vi "ILC Physical Learning.vi"(6 "PID Cluster":T6={"L1 to L4 PID Cluster"={"L1 PID Gains"={"Kp"=0.005, "Kd"=0.5, "Ki"=0.0005}, "L2 PID Gains"={"Kp"=0.01, "Kd"=1.0, "Ki"=0.005}, "L3 PID Gains"={"Kp"=0.05, "Kd"=1.0, "Ki"=0.0005}, "L4 PID Gains"={"Kp"=0.1, "Kd"=0.1, "Ki"=0.0005}}, "Stage PID Cluster"={"Stage Z PID"={"Kp"=0.0005, "Kd"=0.001, "Ki"=0.0}, "Stage Y PID"={"Kp"=0.0003, "Kd"=0.01, "Ki"=0.0}, "Stage X PID"={"Kp"=0.0003, "Kd"=0.01, "Ki"=0.0}}, "OCT Z PID Gains"={"Kp"=0.0003, "Kd"=0.0001, "Ki"=0.01}}, 8 "error in":errorcluster, 9 "Offset Home 2 RCM":dbl[](array[numeric])=[0.0, 0.0, 0.0, 0.0], 10 "Prev Posit Cluster":T5={"Prev L1 to L4 Posit"=[-0.5319, -0.035669172703475985, -2.0566170657346783, 0.9099264705882353], "Prev Stage Posit"=[6.002553885707208, 5.996566124542428, 5.995469940427586], "Prev OCT Z Posit"=-0.0}, 11 "FPGA VI Reference In":refnum<k20>) -> (0 "Eye Model Cluster":T3={"X Grid"=[], "Y Grid"=[], "Za_true Surf"=[], "Iris Center"=[0.0, 5.0, 0.0], "Zp_true Surf"=[], "Pinv"=[[1.0, 0.0], [0.0, 1.0]], "za_true"=0.0, "za_work"=0.0, "zp_work"=0.0, "zp_true"=0.0}, 1 "Trajectory Cluster":T1, 2 "Last Posit Cluster":T4={"Last L1 to L4 Posit"=[0.0, 0.0, 0.0, 0.0], "Last Stage Posit"=[6.0, 6.0, 6.0], "Last OCT Z Posit"=0.0}, 3 "FPGA VI Reference Out":refnum<k20>, 4 "error out":errorcluster, 5 "First Trk Pt":dbl[](array[numeric]))   [LabVIEW 2016]
uses:
  <vilib>/Analysis/Matrix/Datatypes/RealMatrix.ctl
  <vilib>/Platform/TimedLoop/XDataNode/timing_clust.ctl
  <vilib>/Platform/TimedLoop/XDataNode/nitl_modes.ctl
  <vilib>/Platform/TimedLoop/XDataNode/wakeup.ctl
  Global Variables.vi
  <vilib>/platform/TimedLoop/XDataNode/XDataNode.xnode
  <vilib>/Platform/TimedLoop/XDataNode/XDNodeRunTimeDep.lvlib
  <vilib>/Analysis/Matrix/NI_Matrix.lvlib
panel:
  out "In Servo Loop":bool
  out "Loading Finished":bool
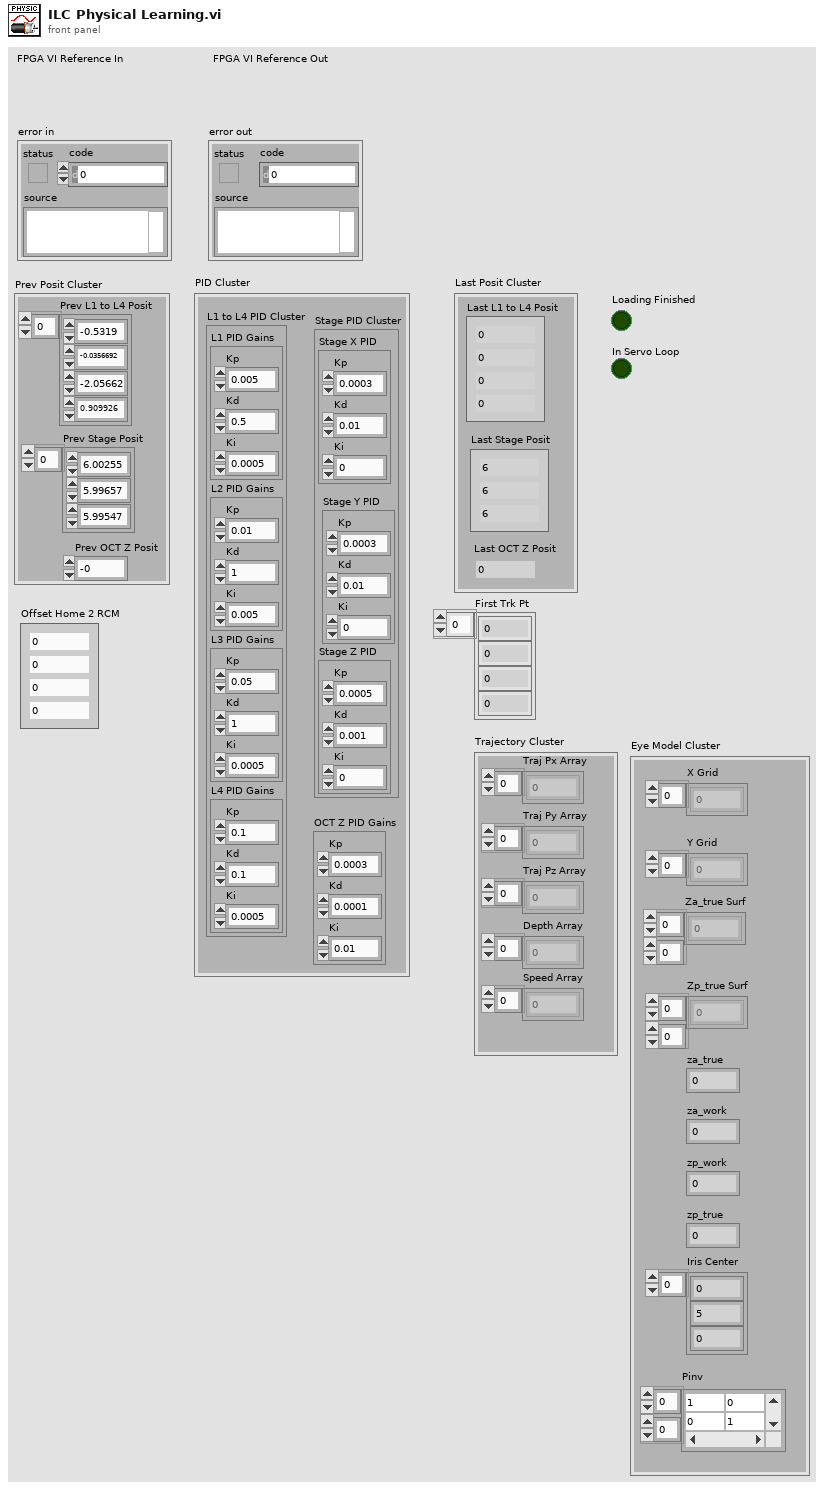
[diagram p1: front panel]
types:
  T1 = cluster{"Traj Px Array":dbl[], "Traj Py Array":dbl[], "Traj Pz Array":dbl[], "Speed Array":dbl[], "Depth Array":dbl[]}
  T2 = typedef "NI_Matrix.lvlib/RealMatrix.ctl" = dbl[][]
  T3 = cluster{"X Grid":dbl[], "Y Grid":dbl[], "Za_true Surf":dbl[][], "Iris Center":dbl[], "Zp_true Surf":dbl[][], "Pinv":T2, "za_true":dbl, "za_work":dbl, "zp_work":dbl, "zp_true":dbl}
  T4 = cluster{"Last L1 to L4 Posit":dbl[], "Last Stage Posit":dbl[], "Last OCT Z Posit":dbl}
  T5 = cluster{"Prev L1 to L4 Posit":dbl[], "Prev Stage Posit":dbl[], "Prev OCT Z Posit":dbl}
  T6 = cluster{"L1 to L4 PID Cluster":cluster{"L1 PID Gains":cluster{"Kp":dbl, "Kd":dbl, "Ki":dbl}, "L2 PID Gains":cluster{"Kp":dbl, "Kd":dbl, "Ki":dbl}, "L3 PID Gains":cluster{"Kp":dbl, "Kd":dbl, "Ki":dbl}, "L4 PID Gains":cluster{"Kp":dbl, "Kd":dbl, "Ki":dbl}}, "Stage PID Cluster":cluster{"Stage Z PID":cluster{"Kp":dbl, "Kd":dbl, "Ki":dbl}, "Stage Y PID":cluster{"Kp":dbl, "Kd":dbl, "Ki":dbl}, "Stage X PID":cluster{"Kp":dbl, "Kd":dbl, "Ki":dbl}}, "OCT Z PID Gains":cluster{"Kp":dbl, "Kd":dbl, "Ki":dbl}}
  T7 = typedef "XDNodeRunTimeDep.lvlib/timing_clust.ctl" = cluster{"Expected End [f-1]":u64, "Actual End [f-1]":u64, "Finished Late? [f-1]":bool, "Expected End [i-1]":u64, "Actual End [i-1]":u64, "Finished Late? [i-1]":bool, "Expected Start [i]":u64, "Actual Start [i]":u64, "Expected Start [f]":u64, "Actual Start [f]":u64, "Source Name":string, "Structure Name":string, "Period":i64, "Deadline":i64, "Offset":i64, "Start":i64, "Priority":i32, "Timeout":i32, "Mode":T8, "Wakeup Reason":T9, "Error":errorcluster, "Source Type":string, "Secondary Source Type":string, "Global End Time":u64, "Global Start Time":u64, "Frame Duration":u64, "Iteration Duration":u64, "Assigned CPU":i32, "I/O Scan Engine Mode":u32}
  T8 = typedef "XDNodeRunTimeDep.lvlib/nitl_modes.ctl" = enum32{"No Change", "Process missed periods, maintain original phase", "Discard missed periods, maintain original phase", "Process missed periods, ignore original phase", "Discard missed periods, ignore original phase"}
  T9 = typedef "XDNodeRunTimeDep.lvlib/wakeup.ctl" = enum32{"Normal", "Aborted", "Asynchronous wakeup", "Timing source error", "Timed loop error", "Timeout"}
  T10 = cluster{"Stop Vacuum":bool, "Vacuum Force":i8, "Max Limit [mmHg]":dbl, "Slide in":i8, "Irrigation?":bool}
  T11 = cluster{"L1 PID Gains":cluster{"Kp":dbl, "Kd":dbl, "Ki":dbl}, "L2 PID Gains":cluster{"Kp":dbl, "Kd":dbl, "Ki":dbl}, "L3 PID Gains":cluster{"Kp":dbl, "Kd":dbl, "Ki":dbl}, "L4 PID Gains":cluster{"Kp":dbl, "Kd":dbl, "Ki":dbl}}
  T12 = cluster{"Stage Z PID":cluster{"Kp":dbl, "Kd":dbl, "Ki":dbl}, "Stage Y PID":cluster{"Kp":dbl, "Kd":dbl, "Ki":dbl}, "Stage X PID":cluster{"Kp":dbl, "Kd":dbl, "Ki":dbl}}
  T13 = cluster{"Accurus button":bool[], "Accurus engaged?":bool, "Vacuum Force":i32, "Accurus Ch. A Vout":dbl, "Accurus Ch. B Vout":dbl, "Irrigation engaged?":bool}
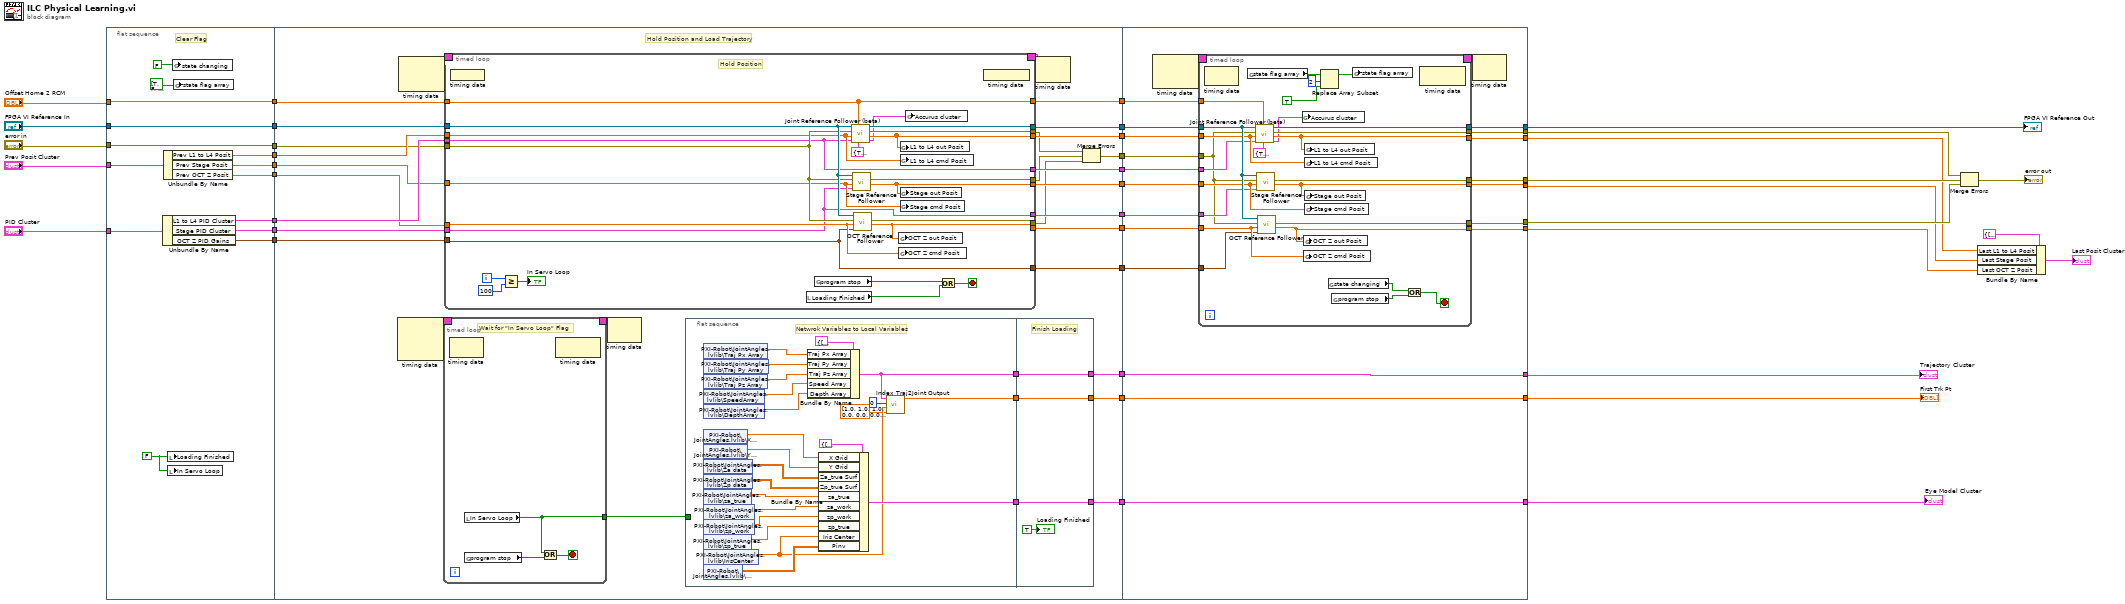
[diagram p0: block diagram]
diagram:
  n1 = flat-sequence {
    tunnel: [w51] -> w39
    tunnel: "FPGA VI Reference In" -> [w51]
    tunnel: [w50] -> w37
    tunnel: "error in" -> [w50]
    tunnel: "Prev Posit Cluster" -> [w49]
    tunnel: "PID Cluster" -> [w48]
    tunnel: [w47] -> w35
    tunnel: [w46] -> w34
    tunnel: "Offset Home 2 RCM" -> [w45]
    tunnel: [w45] -> w32
    tunnel: [w44] -> w29
    tunnel: [w43] -> w28
    tunnel: [w42] -> w27
    tunnel: [w41] -> w26
    tunnel: w39 -> [w68]
    tunnel: w37 -> [w63]
    tunnel: w35 -> [w65]
    tunnel: w34 -> [w64]
    tunnel: w32 -> [w69]
    tunnel: w29 -> [w67]
    tunnel: w28 -> [w62]
    tunnel: w27 -> [w61]
    tunnel: w26 -> [w66]
    tunnel: [w85] -> w13
    tunnel: [w84] -> w12
    tunnel: [w83] -> w11
    tunnel: [w82] -> w10
    tunnel: [w81] -> w9
    tunnel: [w80] -> w8
    tunnel: [w79] -> w7
    tunnel: [w78] -> w6
    tunnel: [w77] -> w5
    tunnel: [w57] -> w4
    tunnel: [w56] -> w3
    tunnel: [w54] -> w2
    tunnel: w13 -> [w165]
    tunnel: [w164] -> w24
    tunnel: [w163] -> w23
    tunnel: [w162] -> w22
    tunnel: w12 -> [w161]
    tunnel: w11 -> [w160]
    tunnel: w10 -> [w159]
    tunnel: w9 -> [w158]
    tunnel: w8 -> [w157]
    tunnel: w7 -> [w156]
    tunnel: w6 -> [w155]
    tunnel: [w154] -> w20
    tunnel: [w153] -> w19
    tunnel: [w152] -> w18
    tunnel: [w151] -> w16
    tunnel: [w148] -> w14
    tunnel: w5 -> [w150]
    tunnel: [w150] -> w15
    tunnel: w4 -> [w149]
    tunnel: w3 -> [w148]
    tunnel: [w147] -> w1
    tunnel: w2 -> [w147]
    frame #0 {
      w40 = FALSE ("Loading Finished")
      # "Clear Flag"
      n2 = Unbundle By Name(w48) -> ("L1 to L4 PID Cluster"=w46:T11, "Stage PID Cluster"=w47:T12, "OCT Z PID Gains"=w41:cluster{"Kp":dbl, "Kd":dbl, "Ki":dbl})
      n3 = Unbundle By Name(w49) -> ("Prev L1 to L4 Posit"=w44:dbl[], "Prev Stage Posit"=w43:dbl[], "Prev OCT Z Posit"=w42:dbl)
      n4 = local write "Loading Finished"(w40) -> ()
      n5 = local write "In Servo Loop"(w40) -> ()
      n6 = global write "Global Variables.vi" "state changing"(FALSE ("state changing")) -> ()
      n7 = global write "Global Variables.vi" "state flag array"(bool[] [TRUE, FALSE, FALSE, FALSE, FALSE, FALSE, FALSE, FALSE, FALSE] ("state flag array")) -> ()
    }
    frame #1 {
      # "Hold Position and Load Trajectory"
      n8 = node-c288() -> (w72:T7)  [unwired: 3 in]
      n9 = node-c288() -> (w76:T7)  [unwired: 2 in]
      n10 = timed-loop {
        timing: w72 -> [_]
        timing-out: [_] -> w71
        tunnel: [w87] -> w70
        stop <- w88 stop-if-true
        # "Wait for \"In Servo Loop\" Flag"
        n11 = node-c288() -> ()  [unwired: 1 in, 1 out]
        n12 = local read "In Servo Loop"() -> (w87:bool)
        n13 = global read "Global Variables.vi" "program stop"() -> (w86:bool)
        n14 = Or(x=w87, y=w86) -> (x .or. y?=w88:bool)
        n15 = node-c288() -> ()  [unwired: 1 in, 1 out]
      }
      n16 = timed-loop {
        timing: w76 -> [_]
        timing-out: [_] -> w75
        tunnel: w67 -> [w136]
        tunnel: w62 -> [w134]
        tunnel: w65 -> [w124]
        tunnel: w64 -> [w125]
        tunnel: w63 -> [w138]
        tunnel: w68 -> [w139]
        tunnel: w69 -> [w131]
        tunnel: w61 -> [w132]
        tunnel: w66 -> [w126]
        tunnel: [w137] -> w83
        tunnel: [w135] -> w82
        tunnel: [w133] -> w81
        tunnel: [w131] -> w84
        tunnel: [w130] -> w85
        tunnel: [w129] -> w60
        tunnel: [w128] -> w59
        tunnel: [w127] -> w58
        tunnel: [w126] -> w80
        tunnel: [w125] -> w79
        tunnel: [w124] -> w78
        i -> [w123]
        stop <- w142 stop-if-true
        # "Hold Position"
        n17 = node-c288 ("Output Node")() -> ()  [unwired: 1 in]
        n18 = Greater Or Equal?(x=w123, y=100) -> (x >= y?=→"In Servo Loop":bool)
        n19 = local read "Loading Finished"() -> (w141:bool)
        n20 = global read "Global Variables.vi" "program stop"() -> (w140:bool)
        n21 = call "Joint Reference Follower (beta).vi"("Accurus Ctrl Cluster"=T10 {"Stop Vacuum"=TRUE, "Vacuum Force"=0, "Max Limit [mmHg]"=600.0, "Slide in"=0, "Irrigation?"=TRUE}, "Offset Home2RCM [deg/mm]"=w131, "PID Ctrl Cluster"=w125, "Ref Array [deg/mm]"=w136, "error in"=w138, "FPGA VI Reference In"=w139) -> ("Accurus Output Cluster"=w119:T13, "Output Posit Array [deg/mm]"=w137:dbl[], "error out"=w129:errorcluster, "FPGA VI Reference Out"=w130:refnum<k20>)  [unwired: 2 in]
        n22 = call "Stage Reference Follower.vi"("Stage PID Cluster"=w124, "Stage cmd Posit [mm]"=w134, "error in"=w138, "FPGA VI Reference In"=w139) -> ("Stage out Posit [mm]"=w135:dbl[], "error out"=w128:errorcluster)  [unwired: 5 in, 1 out]
        n23 = call "OCT Reference Follower.vi"("OCT Z PID Gains"=w126, "OCT  Z cmd Posit [mm]"=w132, "error in"=w138, "FPGA VI Reference In"=w139) -> ("OCT  Z out Posit [mm]"=w133:dbl, "error out"=w127:errorcluster)  [unwired: 5 in, 1 out]
        n24 = global write "Global Variables.vi" "OCT Z out Posit"(w133) -> ()
        n25 = global write "Global Variables.vi" "OCT Z cmd Posit"(w132) -> ()
        n26 = global write "Global Variables.vi" "L1 to L4 out Posit"(w137) -> ()
        n27 = global write "Global Variables.vi" "L1 to L4 cmd Posit"(w136) -> ()
        n28 = global write "Global Variables.vi" "Stage out Posit"(w135) -> ()
        n29 = global write "Global Variables.vi" "Stage cmd Posit"(w134) -> ()
        n30 = global write "Global Variables.vi" "Accurus cluster"(w119) -> ()
        n31 = Or(x=w140, y=w141) -> (x .or. y?=w142:bool)
        n32 = node-c288() -> ()  [unwired: 1 out]
      }
      n33 = node-c288(w71) -> ()  [unwired: 1 out]
      n34 = flat-sequence {
        tunnel: [w98] -> w74
        tunnel: [w96] -> w73
        tunnel: w70 -> [_]
        tunnel: [w93] -> w55
        tunnel: [w117] -> w77
        tunnel: w74 -> [w116]
        tunnel: w73 -> [w117]
        tunnel: [w116] -> w56
        tunnel: [w115] -> w54
        tunnel: w55 -> [w115]
        frame #0 {
          # "Netwrok Variables to Local Variables"
          n35 = shared-variable "PXI-Robot\\JointAngles.lvlib\\Traj Px Array"() -> (w114:dbl[])  [unwired: 1 in, 1 out]
          n36 = shared-variable "PXI-Robot\\JointAngles.lvlib\\Traj Py Array"() -> (w113:dbl[])  [unwired: 1 in, 1 out]
          n37 = shared-variable "PXI-Robot\\JointAngles.lvlib\\Traj Pz Array"() -> (w112:dbl[])  [unwired: 1 in, 1 out]
          n38 = shared-variable "PXI-Robot\\JointAngles.lvlib\\SpeedArray"() -> (w100:dbl[])  [unwired: 1 in, 1 out]
          n39 = shared-variable "PXI-Robot\\JointAngles.lvlib\\DepthArray"() -> (w99:dbl[])  [unwired: 1 in, 1 out]
          n40 = shared-variable "PXI-Robot\\JointAngles.lvlib\\X grid"() -> (w111:dbl[])  [unwired: 1 in, 1 out]
          n41 = shared-variable "PXI-Robot\\JointAngles.lvlib\\Y grid"() -> (w110:dbl[])  [unwired: 1 in, 1 out]
          n42 = shared-variable "PXI-Robot\\JointAngles.lvlib\\Za data"() -> (w109:dbl[][])  [unwired: 1 in, 1 out]
          n43 = shared-variable "PXI-Robot\\JointAngles.lvlib\\Zp data"() -> (w107:dbl[][])  [unwired: 1 in, 1 out]
          n44 = shared-variable "PXI-Robot\\JointAngles.lvlib\\za_true"() -> (w102:dbl)  [unwired: 1 in, 1 out]
          n45 = shared-variable "PXI-Robot\\JointAngles.lvlib\\za_work"() -> (w103:dbl)  [unwired: 1 in, 1 out]
          n46 = shared-variable "PXI-Robot\\JointAngles.lvlib\\zp_work"() -> (w104:dbl)  [unwired: 1 in, 1 out]
          n47 = shared-variable "PXI-Robot\\JointAngles.lvlib\\zp_true"() -> (w105:dbl)  [unwired: 1 in, 1 out]
          n48 = shared-variable "PXI-Robot\\JointAngles.lvlib\\IrisCenter"() -> (w95:dbl[])  [unwired: 1 in, 1 out]
          n49 = shared-variable "PXI-Robot\\JointAngles.lvlib\\Pinv"() -> (w106:T2)  [unwired: 1 in, 1 out]
          n50 = Bundle By Name(cluster=T1 {"Traj Px Array"=[], "Traj Py Array"=[], "Traj Pz Array"=[], "Speed Array"=[], "Depth Array"=[]} ("Trajectory Cluster"), "Traj Px Array"=w114, "Traj Py Array"=w113, "Traj Pz Array"=w112, "Speed Array"=w100, "Depth Array"=w99) -> (w98:T1)
          n51 = Bundle By Name(cluster=T3 {"X Grid"=[], "Y Grid"=[], "Za_true Surf"=[], "Iris Center"=[], "Zp_true Surf"=[], "Pinv"=[], "za_true"=0.0, "za_work"=0.0, "zp_work"=0.0, "zp_true"=0.0} ("Eye Model Cluster"), "X Grid"=w111, "Y Grid"=w110, "Za_true Surf"=w109, "Zp_true Surf"=w107, "za_true"=w102, "za_work"=w103, "zp_work"=w104, "zp_true"=w105, "Iris Center"=w95, "Pinv"=w106) -> (w96:T3)
          n52 = call "Index Traj2Joint Output.vi"("Deform Array"=dbl[] [1.0, 1.0, 1.0, 0.0, 0.0, 0.0, 0.0, 0.0, 0.0], "Pivot Pt"=w95, "Index"=0 ("index"), "Trajectory Cluster"=w98) -> ("Indexed Joit Posit"=w93:dbl[])  [unwired: 6 in, 1 out]
        }
        frame #1 {
          # "Finish Loading"
          "Loading Finished" <- TRUE ("Loading Finished")
        }
      }
      n53 = node-c288(w75) -> ()  [unwired: 1 out]
      n54 = Merge Errors(w60, w59, w58) -> (w57:errorcluster)
    }
    frame #2 {
      n55 = node-c288() -> (w167:T7)  [unwired: 2 in]
      n56 = timed-loop {
        timing: w167 -> [_]
        timing-out: [_] -> w166
        tunnel: w165 -> [w185]
        tunnel: [w184] -> w163
        tunnel: [w183] -> w164
        tunnel: [w182] -> w162
        tunnel: w161 -> [w181]
        tunnel: w160 -> [w180]
        tunnel: w159 -> [w179]
        tunnel: w158 -> [w178]
        tunnel: w157 -> [w177]
        tunnel: w156 -> [w176]
        tunnel: w155 -> [w175]
        tunnel: [w174] -> w154
        tunnel: [w173] -> w153
        tunnel: [w172] -> w152
        tunnel: [w171] -> w151
        tunnel: w149 -> [w170]
        stop <- w192 stop-if-true
        n57 = node-c288() -> ()  [unwired: 1 in, 1 out]
        n58 = global read "Global Variables.vi" "state flag array"() -> (w189:bool[])
        n59 = call "Joint Reference Follower (beta).vi"("Accurus Ctrl Cluster"=T10 {"Stop Vacuum"=TRUE, "Vacuum Force"=0, "Max Limit [mmHg]"=600.0, "Slide in"=0, "Irrigation?"=TRUE}, "Offset Home2RCM [deg/mm]"=w181, "PID Ctrl Cluster"=w176, "Ref Array [deg/mm]"=w180, "error in"=w170, "FPGA VI Reference In"=w185) -> ("Accurus Output Cluster"=w168:T13, "Output Posit Array [deg/mm]"=w174:dbl[], "error out"=w184:errorcluster, "FPGA VI Reference Out"=w171:refnum<k20>)  [unwired: 2 in]
        n60 = call "Stage Reference Follower.vi"("Stage PID Cluster"=w175, "Stage cmd Posit [mm]"=w179, "error in"=w170, "FPGA VI Reference In"=w185) -> ("Stage out Posit [mm]"=w173:dbl[], "error out"=w183:errorcluster)  [unwired: 5 in, 1 out]
        n61 = call "OCT Reference Follower.vi"("OCT Z PID Gains"=w177, "OCT  Z cmd Posit [mm]"=w178, "error in"=w170, "FPGA VI Reference In"=w185) -> ("OCT  Z out Posit [mm]"=w172:dbl, "error out"=w182:errorcluster)  [unwired: 5 in, 1 out]
        n62 = global write "Global Variables.vi" "Accurus cluster"(w168) -> ()
        n63 = global write "Global Variables.vi" "OCT Z out Posit"(w172) -> ()
        n64 = global write "Global Variables.vi" "OCT Z cmd Posit"(w178) -> ()
        n65 = global write "Global Variables.vi" "L1 to L4 out Posit"(w174) -> ()
        n66 = global write "Global Variables.vi" "L1 to L4 cmd Posit"(w180) -> ()
        n67 = global write "Global Variables.vi" "Stage out Posit"(w173) -> ()
        n68 = global write "Global Variables.vi" "Stage cmd Posit"(w179) -> ()
        n69 = Replace Array Subset(array=w189, new element=TRUE ("new element/subarray"), index=2) -> (w188:bool[])
        n70 = global read "Global Variables.vi" "state changing"() -> (w191:bool)
        n71 = global read "Global Variables.vi" "program stop"() -> (w190:bool)
        n72 = global write "Global Variables.vi" "state flag array"(w188) -> ()
        n73 = Or(x=w191, y=w190) -> (x .or. y?=w192:bool)
        n74 = node-c288() -> ()  [unwired: 1 in, 1 out]
      }
      n75 = node-c288(w166) -> ()  [unwired: 1 out]
    }
  }
  n76 = Merge Errors(w23, w24, w22) -> (→"error out":errorcluster)
  n77 = Bundle By Name(cluster=T4 {"Last L1 to L4 Posit"=[0.0, 0.0, 0.0, 0.0], "Last Stage Posit"=[6.0, 6.0, 6.0], "Last OCT Z Posit"=0.0} ("Last Posit Cluster 2"), "Last L1 to L4 Posit"=w20, "Last Stage Posit"=w19, "Last OCT Z Posit"=w18) -> (→"Last Posit Cluster":T4)
  "FPGA VI Reference Out" <- w16
  "First Trk Pt" <- w1
  "Eye Model Cluster" <- w15
  "Trajectory Cluster" <- w14
